vi "Handle S3 Error.vi"(8 "error in (no error)":errorcluster, 9 "Object Path":string, 10 "File Path":path, 11 "Control Experiment in":refnum<class "Control Experiment.lvclass">) -> (0 "error out":errorcluster, 2 "Uploaded to S3":bool, 3 "Control Experiment out":refnum<class "Control Experiment.lvclass">)   [LabVIEW 2016, in "Control Experiment.lvclass"]
uses:
  <userlib>/LevyLab/Transport/Control Experiment/Control Experiment.lvclass
  <vilib>/Utility/sysdir.llb/System Directory Type.ctl
  <userlib>/LevyLab/Transport/Control Experiment/API/S3/S3 Backup--cluster.ctl
  <vilib>/addons/_JKI.lib/Serialization/JSON/JKI JSON Serialization.lvlib
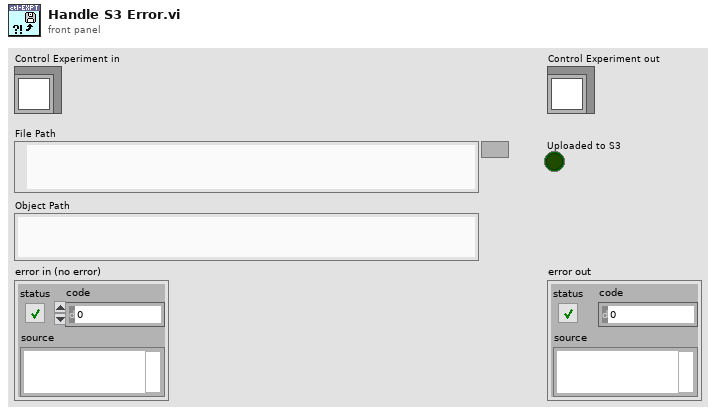
[diagram p1: front panel]
types:
  T1 = typedef "System Directory Type.ctl" = i32
  T2 = enum16{"open", "replace", "create", "open or create", "replace or create", "replace or create with confirmation"}
  T3 = typedef "Control Experiment.lvclass/S3 Backup--cluster.ctl" = cluster{"Time":timestamp, "error":errorcluster, "File Path":path, "Object Path":string}
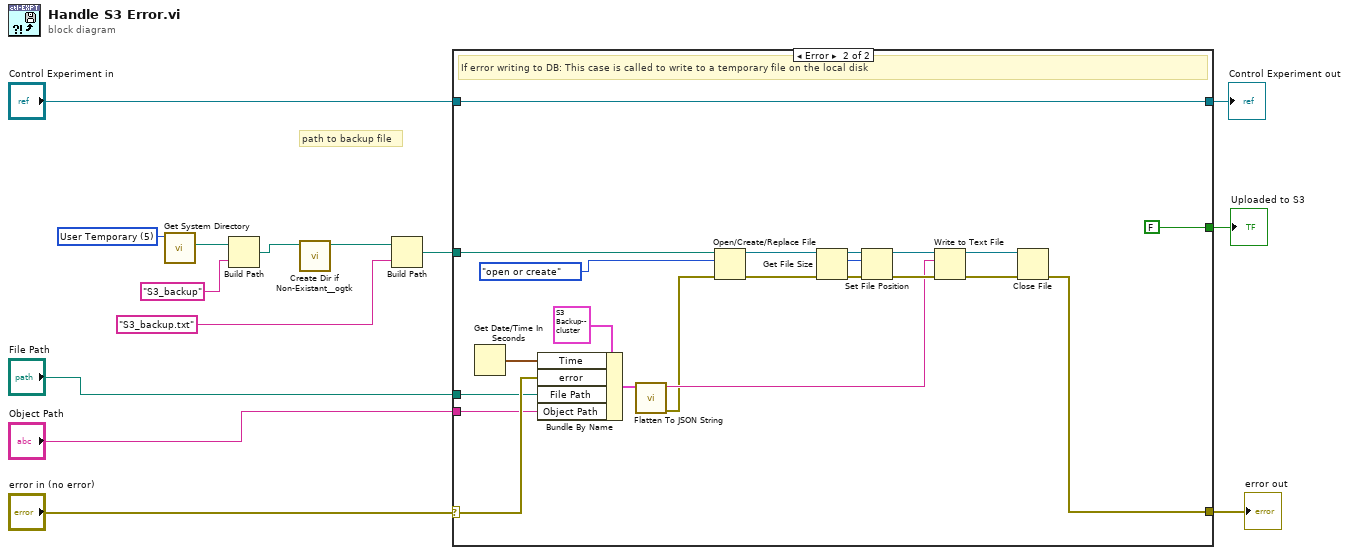
[diagram p0: block diagram]
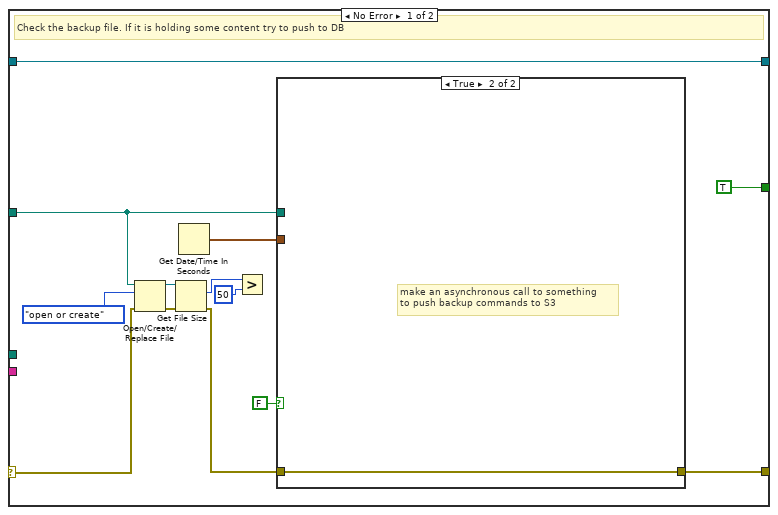
[diagram p2: hidden frame]
diagram:
  w6 = T1 5 items=["User Home"=0, "User Desktop"=1, "User Documents"=2, "User Application Data"=3, "User Preferences"=4, "User Temporary"=5, "Public Documents"=6, "Public Application Data"=7, "Public Preferences"=8, "Public Cache"=13, "System Core Libraries"=9, "System Installed Libraries"=10, "Application Files"=11, "Boot Volume Root"=12] ("system directory type")
  # "path to backup file"
  n1 = call <vilib>:"Get System Directory.vi"("system directory type"=w6) -> ("system directory"=w5:path)  [unwired: 10 in]
  n2 = Build Path(base path=w5, name or relative path="S3_backup") -> (appended path=w3:path)
  n3 = call <userlib>:"Create Dir if Non-Existant__ogtk.vi"("Directory Path"=w3) -> ("dup Directory Path"=w2:path)  [unwired: 8 in, 2 out]
  n4 = Build Path(base path=w2, name or relative path="S3_backup.txt") -> (appended path=w4:path)
  n5 = case shown="Error" "error in (no error)" {
    selector: "error in (no error)" -> [w20 w35]
    tunnel: "Object Path" -> [_ w34]
    tunnel: [TRUE FALSE] -> w9
    tunnel: "Control Experiment in" -> [w16 w38]
    tunnel: w4 -> [w19 w40]
    tunnel: [w21 w39] -> w10
    tunnel: [w16 w38] -> w8
    tunnel: "File Path" -> [_ w33]
    frame No Error {
      # "Check the backup file. If it is holding some content try to push to DB"
      n6 = Open/Create/Replace File(file path (use dialog)=w19, error in=w20, operation (0:open)=T2."open or create") -> (refnum out=w26:refnum<file>, error out=w27:errorcluster)  [unwired: 3 in, 1 out]
      n7 = Get File Size(file=w26, error in=w27) -> (size (in bytes)=w25:i64, 0:w18:errorcluster)  [unwired: 1 out]
      n8 = Get Date/Time In Seconds() -> (seconds since 1Jan1904=w15:timestamp)
      n9 = Greater?(x=w25, y=i64 50) -> ()  [unwired: 1 out]
      n10 = case shown="True" FALSE {
        tunnel: w19 -> [_ _]
        tunnel: [w28 w29] -> w21
        tunnel: w18 -> [w28 w29]
        tunnel: w15 -> [_ _]
        frame False {
        }
        frame True {
          # "make an asynchronous call to something\nto push backup commands to S3"
        }
      }
    }
    frame Error {
      # "If error writing to DB: This case is called to write to a temporary file on the local disk"
      n11 = Get Date/Time In Seconds() -> (seconds since 1Jan1904=w36:timestamp)
      n12 = Bundle By Name(cluster=T3 {"Time"=timestamp(0 s since 1904-01-01), "error"={"status"=FALSE, "code"=0, "source"=""}, "File Path"=path "", "Object Path"=""} ("S3 Backup"), "Time"=w36, "error"=w35, "File Path"=w33, "Object Path"=w34) -> (w31:T3)
      n13 = call <vilib>:"Flatten To JSON String.vi"("Variant"=w31) -> ("error out"=w30:errorcluster, "JSON String"=w37:string)  [unwired: 9 in]
      n14 = Open/Create/Replace File(file path (use dialog)=w40, error in=w30, operation (0:open)=T2."open or create") -> (refnum out=w43:refnum<file>, error out=w42:errorcluster)  [unwired: 3 in, 1 out]
      n15 = Get File Size(file=w43, error in=w42) -> (refnum out=w49:refnum<file>, size (in bytes)=w50:i64, 0:w51:errorcluster)
      n16 = Set File Position(offset (in bytes) (0)=w50, refnum=w49, error in=w51) -> (refnum out=w47:refnum<file>, error out=w48:errorcluster)  [unwired: 1 in]
      n17 = Write to Text File(file (use dialog)=w47, text=w37, error in=w48) -> (refnum out=w45:refnum<file>, error out=w46:errorcluster)  [unwired: 1 in, 1 out]
      n18 = Close File(refnum=w45, error in=w46) -> (error out=w39:errorcluster)  [unwired: 1 out]
    }
  }
  "error out" <- w10
  "Uploaded to S3" <- w9
  "Control Experiment out" <- w8
